vi "Seconds Breakdown.vi"(10 "Total Time in Seconds":dbl) -> (1 "Seconds":dbl, 2 "Minutes":dbl, 3 "Hours":dbl)   [LabVIEW 2014]
doc: "This VI converts seconds into hours, minutes, and seconds.\n\nInput: Total Time in Seconds\nOutputs: Seconds, Minutes, Hours\n\nDivide seconds by 3600; quotient is the number of hours, remainder is remaining number of seconds.\nDivide remaining number of seconds by 60; quotient is the number of minutes, remaider is number of seconds."
panel:
  # "Connector Pane ^"
  # "^ \nRun Button"
  # "Icon ^"
  # "Converts seconds into a combination of hours, minutes and seconds."
  # "Indicator"
  # "Control"
  # "Indicator"
  # "Indicator"
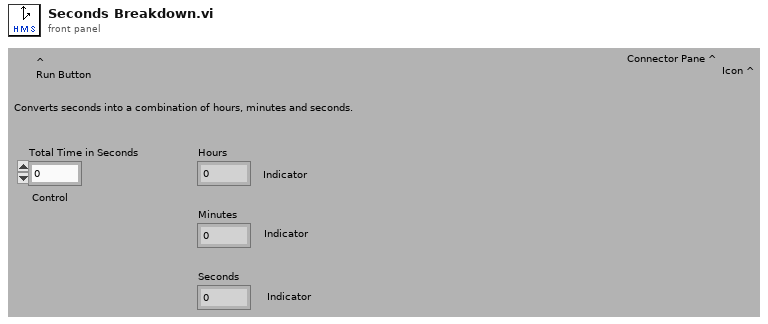
[diagram p1: front panel]
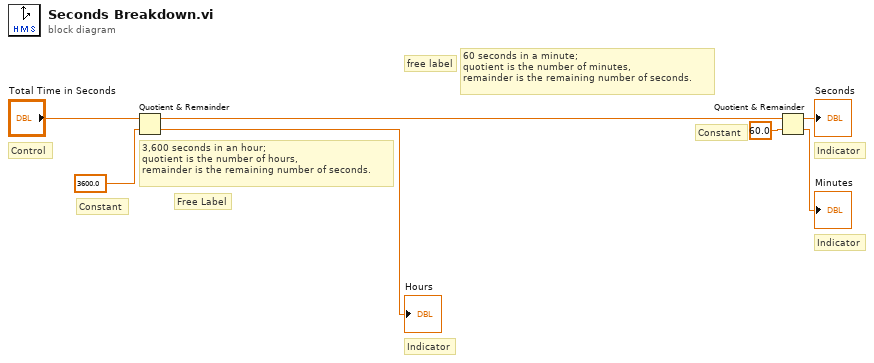
[diagram p0: block diagram]
diagram:
  # "Constant"
  # "Constant"
  # "Control"
  # "Indicator"
  # "Indicator"
  # "Indicator"
  # "Free Label"
  # "free label"
  # "60 seconds in a minute;\nquotient is the number of minutes,\nremainder is the remaining number of seconds."
  # "3,600 seconds in an hour;\nquotient is the number of hours, \nremainder is the remaining number of seconds."
  n1 = Quotient & Remainder(x="Total Time in Seconds", y=3600.0) -> (x-y*floor(x/y)=w4:dbl, floor(x/y)=→"Hours":dbl)
  n2 = Quotient & Remainder(x=w4, y=60.0) -> (x-y*floor(x/y)=→"Seconds":dbl, floor(x/y)=→"Minutes":dbl)
